vi "Example QR Code.vi"() -> ()   [LabVIEW 2020]
uses:
  g_ar_toolkit.image/g_ar_toolkit.image.lvlib
  g_ar_toolkit.image/ARGB Colour.ctl
  g_ar_toolkit.image/Font Face.ctl
  g_ar_toolkit.image/Text Drawing Settings.ctl
  g_ar_toolkit.feature_detection/QR Code Detector/QR Code Detector.lvclass
  g_ar_toolkit.image/New Image (ARGB).vi
  g_ar_toolkit.image/Read Image File (ARGB).vi
  g_ar_toolkit.image/Draw Image to Picture (ARGB).vi
  g_ar_toolkit.image/Draw Poly Lines (ARGB).vi
  g_ar_toolkit.image/Draw Text (ARGB).vi
  g_ar_toolkit.feature_detection/QR Code Detector/Detect QR Codes (ARGB).vi
  g_ar_toolkit.feature_detection/QR Code Detector/Detection.ctl
  g_ar_toolkit.common/Image Point (Float).ctl
  g_ar_toolkit.common/g_ar_toolkit.common.lvlib
  g_ar_toolkit.feature_detection/QR Code Detector/Detection Region.ctl
panel:
  out "Detections":T1[](array[typedef])
  out "Picture":picture
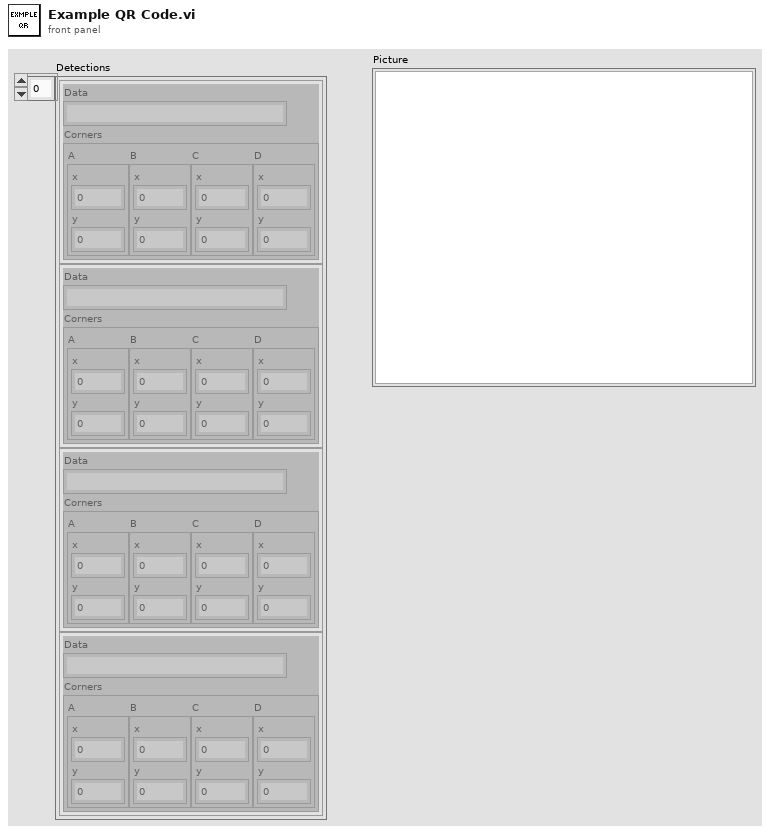
[diagram p1: front panel]
types:
  T1 = typedef "g_ar_toolkit.feature_detection.lvlib/QR Code Detector.lvclass/Detection.ctl" = cluster{"Data":string, "Corners":T2}
  T2 = typedef "g_ar_toolkit.feature_detection.lvlib/QR Code Detector.lvclass/Detection Region.ctl" = cluster{"A":T3, "B":T3, "C":T3, "D":T3}
  T3 = typedef "g_ar_toolkit.common.lvlib/Image Point (Float).ctl" = cluster{"x":dbl, "y":dbl}
  T4 = typedef "g_ar_toolkit.image.lvlib/ARGB Image.ctl" = refnum<data-value>
  T5 = typedef "g_ar_toolkit.image.lvlib/Text Drawing Settings.ctl" = cluster{"OpenCV Font Face":T6, "Font Scale":dbl}
  T6 = typedef "g_ar_toolkit.image.lvlib/Font Face.ctl" = enum8{"FONT_HERSHEY_SIMPLEX", "FONT_HERSHEY_PLAIN", "FONT_HERSHEY_DUPLEX", "FONT_HERSHEY_COMPLEX", "FONT_HERSHEY_TRIPLEX", "FONT_HERSHEY_COMPLEX_SMALL", "FONT_HERSHEY_SCRIPT_SIMPLEX", "FONT_HERSHEY_SCRIPT_COMPLEX", "FONT_ITALIC"}
  T7 = typedef "g_ar_toolkit.image.lvlib/ARGB Colour.ctl" = cluster{"Alpha":u8, "RGB":u32}
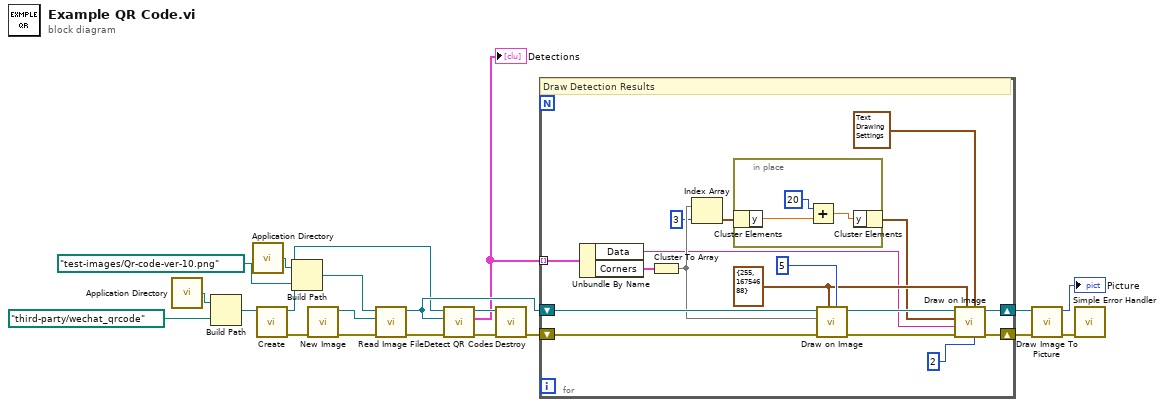
[diagram p0: block diagram]
diagram:
  n1 = call <vilib>:"Application Directory.vi"() -> ("Application Directory"=w15:path)
  n2 = Build Path(base path=w15, name or relative path=path "third-party/wechat_qrcode" ("Filepath")) -> (appended path=w3:path)
  n3 = call <vilib>:"Application Directory.vi"() -> ("Application Directory"=w18:path)
  n4 = call "Create.vi"("Model Directory"=w3) -> ("error out"=w1:errorcluster, "New QR Code Detector"=w2:refnum<class "QR Code Detector.lvclass">)  [unwired: 9 in]
  n5 = Build Path(base path=w18, name or relative path=path "test-images/Qr-code-ver-10.png" ("Path")) -> (appended path=w17:path)
  n6 = call-poly "New Image.vi"("error in (no error)"=w1) -> ("error out"=w14:errorcluster, "New ARGB Image"=w20:T4)  [unwired: 9 in]
  n7 = call-poly "Read Image File.vi"("error in (no error)"=w14, "ARGB Image Destination"=w20, "Filepath"=w17) -> ("error out"=w4:errorcluster, "ARGB Image Destination (duplicate)"=w11:T4)  [unwired: 7 in]
  n8 = call-poly "Detect QR Codes.vi"("error in (no error)"=w4, "ARGB Image"=w11, "QR Code Detector in"=w2) -> ("error out"=w12:errorcluster, "Detections"=w10:T1[], "QR Code Detector (Duplicate)"=w13:refnum<class "QR Code Detector.lvclass">)  [unwired: 6 in]
  "Detections" <- w10
  n9 = call "Destroy.vi"("error in (no error)"=w12, "QR Code Detector in"=w13) -> ("error out"=w9:errorcluster)  [unwired: 9 in]
  n10 = for {
    shift-right: [w29] -> w7
    shift-left: w11 -> [w37]
    tunnel: w10 -> [w36] mode=indexing
    shift-right: [w31] -> w8
    shift-left: w9 -> [w34]
    w28 = T7 {"Alpha"=255, "RGB"=16754688} ("ARGB Colour")
    # "Draw Detection Results"
    n11 = Unbundle By Name(w36) -> ("Data"=w22:string, "Corners"=w35:T2)
    n12 = Cluster To Array(cluster=w35) -> (array=w27:T3[])
    n13 = Index Array(array=w27, index=3) -> (element=w25:T3)
    n14 = in-place {
      n15 = in-place-cluster #1(w25) -> ("y"=w40:dbl)
      n16 = Add(x=20, y=w40) -> (x+y=w39:dbl)
      n17 = in-place-cluster #1("y"=w39) -> (w24:T3)
    }
    n18 = call-poly "Draw on Image.vi"("Thickness (Default: 1)"=5, "ARGB Colour"=w28, "error in (no error)"=w34, "Points"=w27, "ARGB Image"=w37) -> ("error out"=w33:errorcluster, "ARGB Image (Duplicate)"=w30:T4)  [unwired: 5 in]
    n19 = call-poly "Draw on Image.vi"("Thickness (Default: 1)"=2, "Text Drawing Settings (Default: Simplex)"=T5 {"OpenCV Font Face"=enum."FONT_HERSHEY_SIMPLEX", "Font Scale"=0.6}, "ARGB Colour"=w28, "error in (no error)"=w33, "Text"=w22, "Origin"=w24, "ARGB Image"=w30) -> ("error out"=w31:errorcluster, "ARGB Image (Duplicate)"=w29:T4)  [unwired: 3 in]
  }
  n20 = call-poly "Draw Image To Picture.vi"("error in (no error)"=w8, "ARGB Image Source"=w7) -> ("error out"=w6:errorcluster, "Picture"=→"Picture":picture)  [unwired: 8 in]
  n21 = call <vilib>:"Simple Error Handler.vi"("error in (no error)"=w6) -> ()  [unwired: 4 in, 5 out]
